vi "HAPS_LoadTable_SetBeam_Manual_Selected_Two_Phase.vi"() -> ()   [LabVIEW 2023, in "HAPS.lvlib"]
uses:
  HAPS.lvlib
  set_ele.ctl
  HAPS_SerialPort.ctl
  HAPS_MCU_ELE_Func.ctl
  <vilib>/Utility/file.llb/Read Delimited Spreadsheet (string).vi
  R_S/R_S.lvlib
panel:
  in  "Phase_offset?":i32
  in  "ele_gain_2":i32=35
  in  "BFIC_id_2?":i32
  in  "Group_2?":i32
  in  "ele_gain_1":i32=35
  in  "BFIC_id_1?":i32
  in  "Group_1?":i32
  in  "sys reboot?":bool=TRUE
  in  "VISA resource name":refnum<visa-resource-name>="COM1"
  in  "file path":path=path "D:/_Project/_Code/LabVIEW/_CLC_Gen4/CLC_LV2023/CLC_Cali/Log/HAPS/Preset.csv"
  out "error IO":errorcluster
  out "Err_code":i32
  out "status":bool
  in  "simu.?":bool
  in  "set_ele":T1={"ch"=0, "chain_id"=0, "group"=0, "array_id"=0, "ele_phase"=0, "ele_gain"=35, "com_gain"=17, "pd_range"=0}
  out "ele phase":i32
  out "ele gain":i32
  out "channel":i32
  out "chain ID":i32
  out "group":i32
  out "array id":i32
  # "HAPS 24x24 Setting Manual In-Phase : \n                                           Two BFIC Phase"
  # "Tx:35\nRx:22"
  # "Not using!!!!!!!!!!!!!!!!!!!!!!!!!!!!!!!!!!!!!!!!"
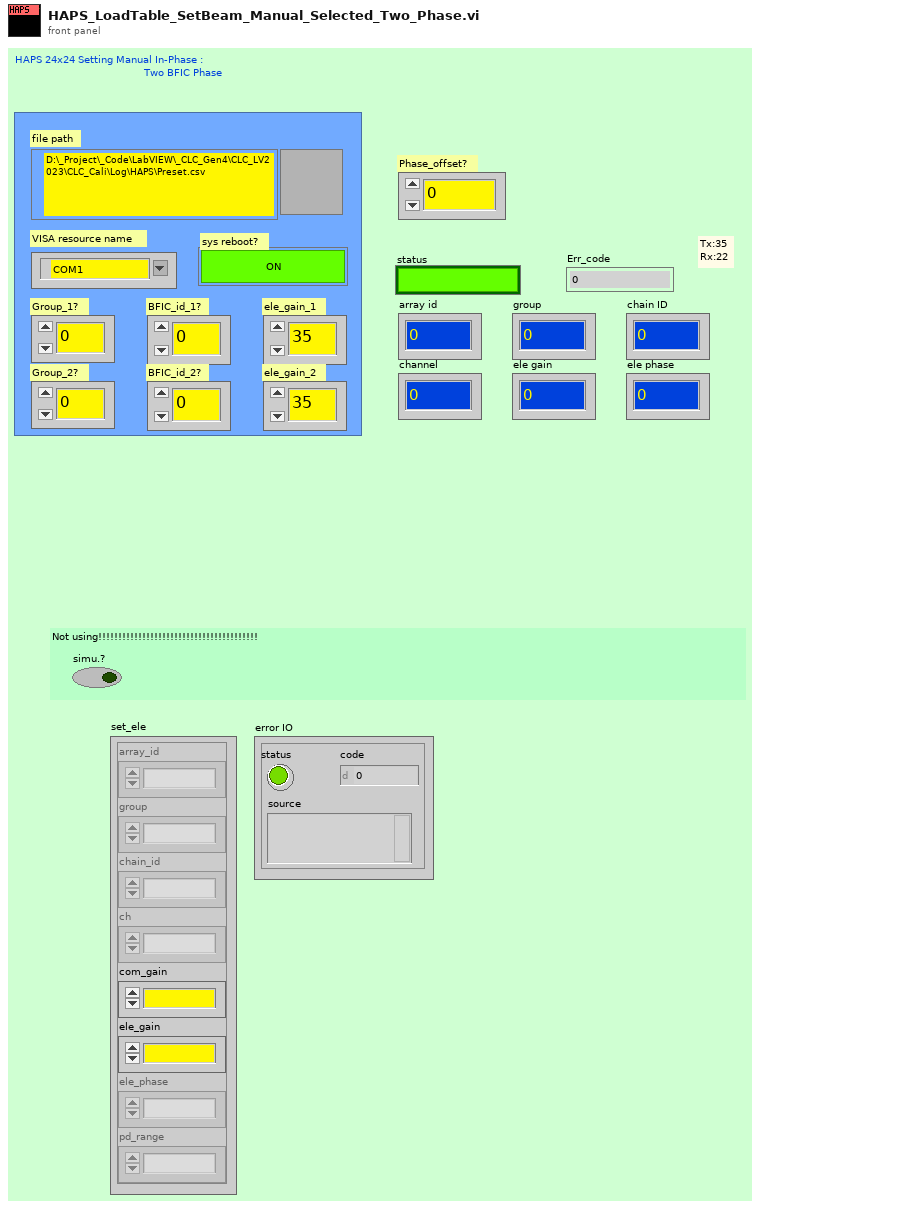
[diagram p1: front panel]
types:
  T1 = typedef "HAPS.lvlib/set_ele.ctl" = cluster{"ch":i32, "chain_id":i32, "group":i32, "array_id":i32, "ele_phase":i32, "ele_gain":i32, "com_gain":i32, "pd_range":i32}
  T2 = typedef "HAPS.lvlib/HAPS_SerialPort.ctl" = enum16{"Init", "Close", "CMD", "Flush"}
  T3 = typedef "HAPS.lvlib/HAPS_MCU_ELE_Func.ctl" = enum16{"array_init", "set_com_gain", "set_ch_gain_phase", "set_pd_range", "get_preamp_temp", "get_bfic_temp", "get_tx_pd", "ch_on", "ch_on_2", "ch_ctrl_all", "array_ctrl_src"}
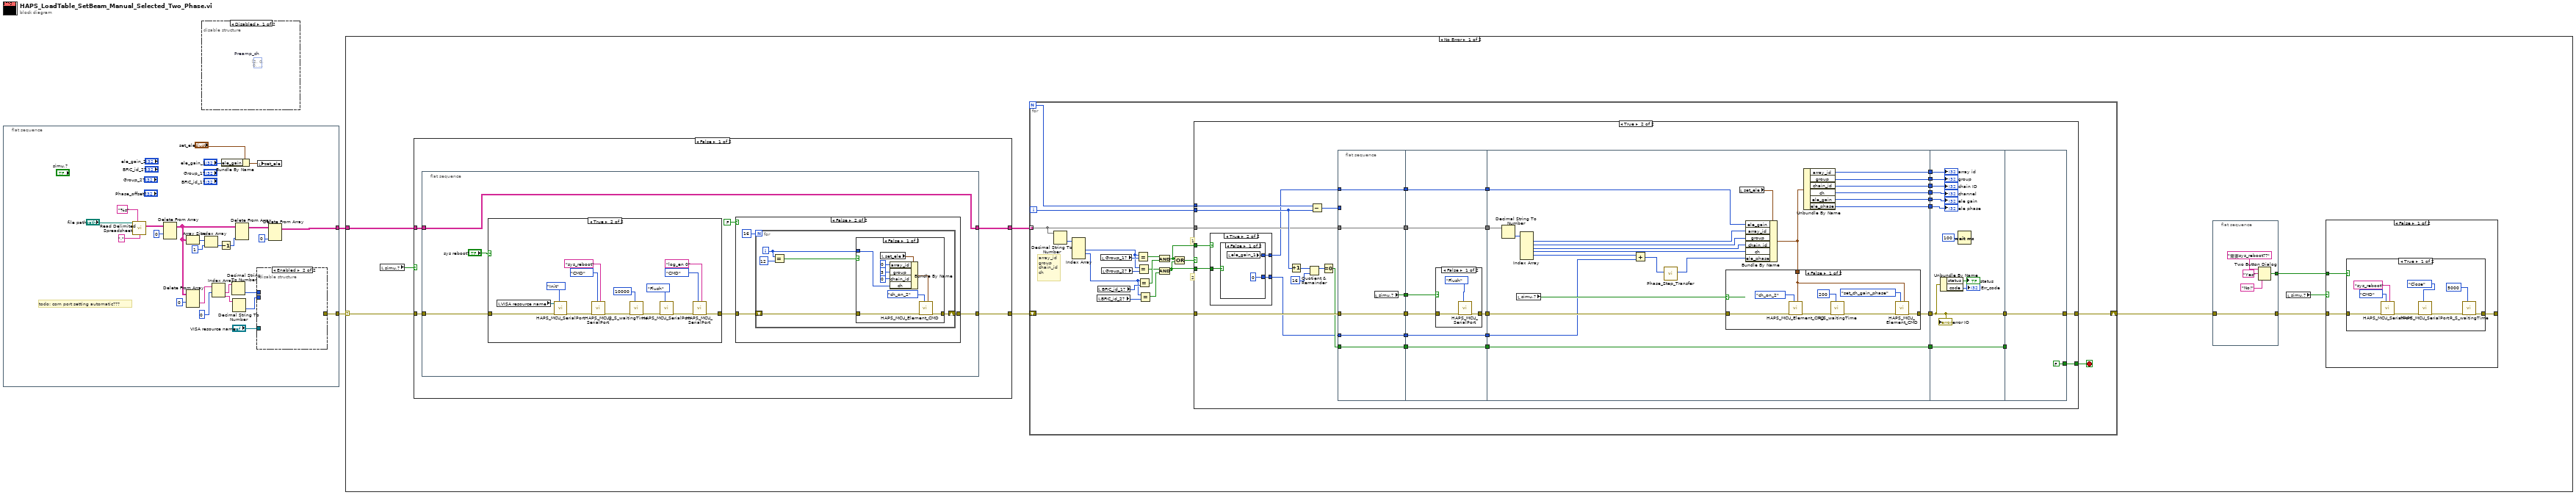
[diagram p0: block diagram]
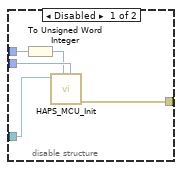
[diagram p2: hidden frame]
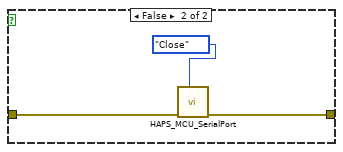
[diagram p4: hidden frame]
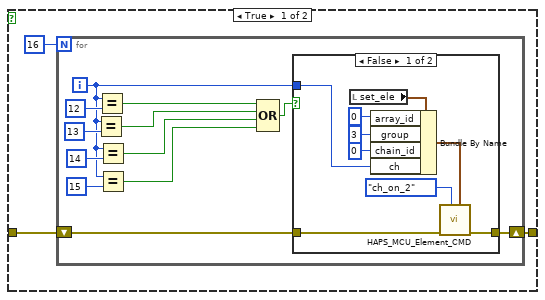
[diagram p6: hidden frame]
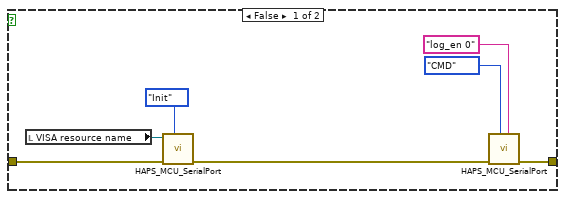
[diagram p9: hidden frame]
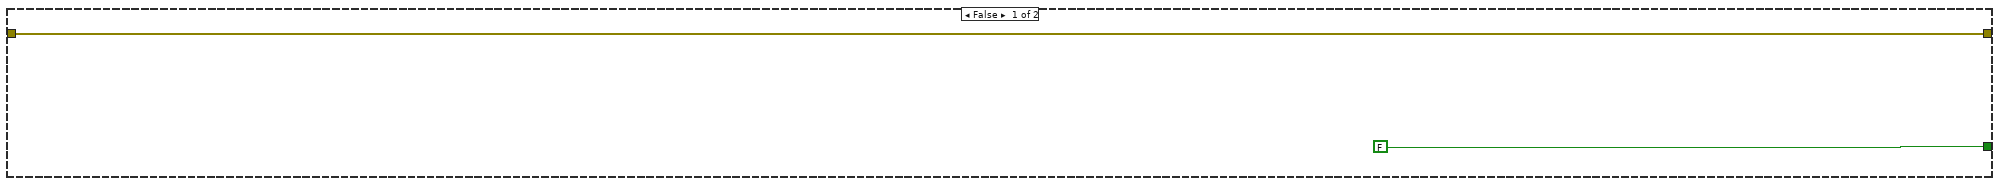
[diagram p11: hidden frame]
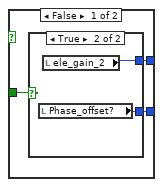
[diagram p12: hidden frame]
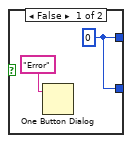
[diagram p13: hidden frame]
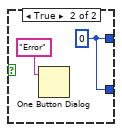
[diagram p14: hidden frame]
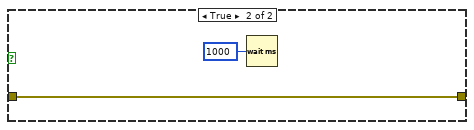
[diagram p16: hidden frame]
diagram:
  n1 = flat-sequence {
    tunnel: [w19] -> w2
    tunnel: [w6] -> w1
    frame #0 {
      # "todo: com port setting automatic???"
      n2 = call-poly <vilib>:"Read Delimited Spreadsheet.vi"("file path (dialog if empty)"="file path", "format (%s)"="%s" ("format (%.3f)"), "delimiter (\\t)"="," ("delimiter (\\t)")) -> ("all rows"=w25:string[][])  [unwired: 7 in, 5 out]
      n3 = Delete From Array(array=w25, index (row)=0) -> (array with subset deleted=w15:string[][])  [unwired: 2 in, 1 out]
      n4 = Array Size(array=w15) -> (size(s)=w23:i32[])
      n5 = Delete From Array(array=w15, index (row)=0) -> (deleted portion=w14:string[])  [unwired: 2 in, 1 out]
      n6 = Index Array(array=w23, index=1) -> (element=w20:i32)
      n7 = Index Array(array=w14, index #1=0 ("index")) -> (element #1=w13:string, element #2=w12:string)  [unwired: 1 in]
      n8 = Decrement(x=w20) -> (x-1=w22:i32)
      n9 = Bundle By Name(cluster="set_ele", "ele_gain"="ele_gain_1") -> (w3:T1)
      n10 = Decimal String To Number(string=w13) -> (number=w9:i32)  [unwired: 2 in, 1 out]
      n11 = Decimal String To Number(string=w12) -> (number=w8:i32)  [unwired: 2 in, 1 out]
      n12 = Delete From Array(array=w15, index (col)=w22) -> (array with subset deleted=w18:string[][])  [unwired: 2 in, 1 out]
      n13 = disable-structure shown="Enabled" {
        disable-tunnel: [w32 _] -> w19
        disable-tunnel: w9 -> [w31 _]
        disable-tunnel: w8 -> [w30 _]
        disable-tunnel: "VISA resource name" -> [w29 _]
        frame Disabled {
          n14 = To Unsigned Word Integer(number=w31) -> (unsigned 16bit integer=w28:u16)
          n15 = call "HAPS_MCU_Init.vi"("array_id"=w30, "Tx/Rx"=w28, "VISA resource name"=w29) -> ("error out"=w32:errorcluster)  [unwired: 8 in]
        }
        frame Enabled {
        }
      }
      n16 = local write "set_ele"(w3) -> ()
      n17 = Delete From Array(array=w18, index (col)=0 ("index (row)")) -> (array with subset deleted=w6:string[][])  [unwired: 2 in, 1 out]
    }
  }
  n18 = disable-structure shown="Disabled" {
    frame Disabled {
      (unwired) i32[][] [[2, 0, 0, 8, 8, 10, 11, 9, 9, 1, 1, 3], [3, 1, 1, 9, 9, 11, 13, 15, 15, 7, 7, 5], [5, 7, 7, 15, 15, 13, 14, 14, 6, 6, 4, 12]]  # Preamp_ch
    }
    frame Enabled {
    }
  }
  n19 = case shown="No Error" w2 {
    selector: w2 -> [w39 _]
    tunnel: w1 -> [w41 _]
    frame No Error {
      n20 = local read "simu.?"() -> (w37:bool)
      n21 = case shown="False" w37 {
        tunnel: w41 -> [w65 w137]
        tunnel: [w64 w137] -> w40
        tunnel: w39 -> [w63 w136]
        tunnel: [w62 w136] -> w38
        frame False {
          n22 = flat-sequence {
            tunnel: w65 -> [w71]
            tunnel: [w71] -> w64
            tunnel: w63 -> [w69]
            tunnel: [w70] -> w62
            frame #0 {
              n23 = case shown="True" "sys reboot?" {
                tunnel: w69 -> [w119 w133]
                tunnel: [w117 w131] -> w68
                frame False {
                  n24 = local read "VISA resource name"() -> (w115:refnum<visa-resource-name>)
                  n25 = call "HAPS_MCU_SerialPort.vi"("HAPS_SerialPort_Func"=HAPS_SerialPort."Init", "error in"=w119, "VISA resource name"=w115) -> ("error out"=w116:errorcluster)  [unwired: 6 in, 2 out]
                  n26 = call "HAPS_MCU_SerialPort.vi"("Command"="log_en 0", "HAPS_SerialPort_Func"=enum16{"Init", "Close", "CMD"}."CMD" ("HAPS_SerialPort"), "error in"=w116) -> ("error out"=w117:errorcluster)  [unwired: 6 in, 2 out]
                }
                frame True {
                  n27 = local read "VISA resource name"() -> (w122:refnum<visa-resource-name>)
                  n28 = call "HAPS_MCU_SerialPort.vi"("HAPS_SerialPort_Func"=HAPS_SerialPort."Init", "error in"=w133, "VISA resource name"=w122) -> ("error out"=w128:errorcluster)  [unwired: 6 in, 2 out]
                  n29 = call "HAPS_MCU_SerialPort.vi"("Command"="sys_reboot", "HAPS_SerialPort_Func"=enum16{"Init", "Close", "CMD"}."CMD" ("HAPS_SerialPort"), "error in"=w128) -> ("error out"=w127:errorcluster)  [unwired: 6 in, 2 out]
                  n30 = call "R_S_waitingTime.vi"("Waiting Time(ms)"=u32 10000, "error in"=w127) -> ("error out"=w125:errorcluster)  [unwired: 9 in]
                  n31 = call "HAPS_MCU_SerialPort.vi"("HAPS_SerialPort_Func"=HAPS_SerialPort."Flush", "error in"=w125) -> ("error out"=w123:errorcluster)  [unwired: 7 in, 2 out]
                  n32 = call "HAPS_MCU_SerialPort.vi"("Command"="log_en 0", "HAPS_SerialPort_Func"=enum16{"Init", "Close", "CMD"}."CMD" ("HAPS_SerialPort"), "error in"=w123) -> ("error out"=w131:errorcluster)  [unwired: 6 in, 2 out]
                }
              }
              n33 = case shown="False" FALSE {
                tunnel: [w73 w98] -> w70
                tunnel: w68 -> [w72 w97]
                frame True {
                  n34 = for {
                    N: 16 -> [_]
                    shift-right: [w85] -> w73
                    shift-left: w72 -> [w86]
                    i -> [w76]
                    n35 = Equal?(x=w76, y=13) -> (x = y?=w80:bool)
                    n36 = Equal?(x=w76, y=12) -> (x = y?=w84:bool)
                    n37 = Equal?(x=w76, y=14) -> (x = y?=w78:bool)
                    n38 = Equal?(x=w76, y=15) -> (x = y?=w75:bool)
                    n39 = Compound Arithmetic op=OR(w84, w80, w78, w75) -> (w81:bool)
                    n40 = case shown="False" w81 {
                      tunnel: w86 -> [w89 w96]
                      tunnel: [w88 w96] -> w85
                      tunnel: w76 -> [w87 _]
                      frame False {
                        n41 = local read "set_ele"() -> (w91:T1)
                        n42 = Bundle By Name(cluster=w91, "array_id"=0, "group"=3, "chain_id"=0, "ch"=w87) -> (w92:T1)
                        n43 = call "HAPS_MCU_Element_CMD.vi"("set_ele"=w92, "HAPS_MCU_ELE_Func."=HAPS_MCU_ELE_Func."ch_on_2", "error in"=w89) -> ("error out"=w88:errorcluster)  [unwired: 7 in, 1 out]
                      }
                      frame True {
                      }
                    }
                  }
                }
                frame False {
                  n44 = for {
                    N: 16 -> [_]
                    shift-right: [w103] -> w98
                    shift-left: w97 -> [w104]
                    i -> [w101]
                    n45 = Equal?(x=w101, y=12) -> (x = y?=w100:bool)
                    n46 = case shown="False" w100 {
                      tunnel: w104 -> [w107 w114]
                      tunnel: [w106 w114] -> w103
                      tunnel: w101 -> [w105 _]
                      frame False {
                        n47 = local read "set_ele"() -> (w109:T1)
                        n48 = Bundle By Name(cluster=w109, "array_id"=0, "group"=3, "chain_id"=0, "ch"=w105) -> (w110:T1)
                        n49 = call "HAPS_MCU_Element_CMD.vi"("set_ele"=w110, "HAPS_MCU_ELE_Func."=HAPS_MCU_ELE_Func."ch_on_2", "error in"=w107) -> ("error out"=w106:errorcluster)  [unwired: 7 in, 1 out]
                      }
                      frame True {
                      }
                    }
                  }
                }
              }
            }
          }
        }
        frame True {
        }
      }
      n50 = for {
        N -> [w155]
        tunnel: w40 -> [w152] mode=indexing
        shift-right: [w157] -> w34
        shift-left: w38 -> [w156]
        i -> [w154]
        stop <- w151 stop-if-true
        # "2"
        # "1"
        # "array_id\ngroup\nchain_id\nch"
        n51 = Decimal String To Number(string=w152) -> (number=w153:i32[])  [unwired: 2 in, 1 out]
        n52 = Index Array(array=w153) -> (element #2=w147:i32, element #3=w144:i32)  [unwired: 4 in, 2 out]
        n53 = local read "BFIC_id_2?"() -> (w143:i32)
        n54 = local read "BFIC_id_1?"() -> (w145:i32)
        n55 = local read "Group_1?"() -> (w148:i32)
        n56 = local read "Group_2?"() -> (w146:i32)
        n57 = Equal?(x=w147, y=w148) -> (x = y?=w150:bool)
        n58 = Equal?(x=w147, y=w146) -> (x = y?=w142:bool)
        n59 = Equal?(x=w144, y=w145) -> (x = y?=w149:bool)
        n60 = Equal?(x=w144, y=w143) -> (x = y?=w141:bool)
        n61 = Compound Arithmetic op=AND(w150, w149) -> (w139:bool)
        n62 = Compound Arithmetic op=AND(w142, w141) -> (w138:bool)
        n63 = Compound Arithmetic op=OR(w139, w138) -> (w140:bool)
        n64 = case shown="True" w140 {
          tunnel: [w158 w179] -> w157
          tunnel: w156 -> [w158 w178]
          tunnel: w155 -> [_ w177]
          tunnel: w154 -> [_ w176]
          tunnel: w152 -> [_ w175]
          tunnel: [FALSE ("T button?") w169] -> w151
          tunnel: w139 -> [_ w167]
          tunnel: w138 -> [_ w166]
          frame False {
          }
          frame True {
            n65 = case shown="True" w167 {
              tunnel: w166 -> [w198 w204]
              tunnel: [w197 w205] -> w163
              tunnel: [w196 w203] -> w160
              frame False {
                n66 = case shown="True" w198 {
                  tunnel: [w199 w202] -> w197
                  tunnel: [w199 w201] -> w196
                  frame False {
                    w199 = 0 ("ele_gain_2")
                    n67 = One Button Dialog(message="Error") -> ()  [unwired: 1 in, 1 out]
                  }
                  frame True {
                    n68 = local read "Phase_offset?"() -> (w201:i32)
                    n69 = local read "ele_gain_2"() -> (w202:i32)
                  }
                }
              }
              frame True {
                n70 = case shown="False" w204 {
                  tunnel: [w207 w208] -> w205
                  tunnel: [0 ("ele_gain_2") w208] -> w203
                  frame False {
                    n71 = local read "ele_gain_1"() -> (w207:i32)
                  }
                  frame True {
                    w208 = 0 ("ele_gain_1")
                    n72 = One Button Dialog(message="Error") -> ()  [unwired: 1 in, 1 out]
                  }
                }
              }
            }
            n73 = Increment(x=w176) -> (x+1=w173:i32)
            n74 = Quotient & Remainder(x=w173, y=16) -> (x-y*floor(x/y)=w171:i32)  [unwired: 1 out]
            n75 = Subtract(x=w177, y=w176) -> (x-y=w174:i32)
            n76 = Equal To 0?(x=w171) -> (x = 0?=w170:bool)
            n77 = flat-sequence {
              tunnel: w174 -> [_]
              tunnel: w178 -> [w214]
              tunnel: w175 -> [w215]
              tunnel: [w215] -> w195
              tunnel: [w214] -> w194
              tunnel: w170 -> [w213]
              tunnel: [w213] -> w193
              tunnel: [w212] -> w168
              tunnel: [w211] -> w164
              tunnel: w163 -> [w211]
              tunnel: [w210] -> w161
              tunnel: w160 -> [w210]
              tunnel: [w222] -> w192
              tunnel: [w221] -> w191
              tunnel: w195 -> [w222]
              tunnel: w194 -> [w220]
              tunnel: w193 -> [w219]
              tunnel: [w219] -> w190
              tunnel: w168 -> [w218]
              tunnel: [w217] -> w165
              tunnel: w164 -> [w217]
              tunnel: [w216] -> w162
              tunnel: w161 -> [w216]
              tunnel: w192 -> [w249]
              tunnel: w191 -> [w247]
              tunnel: [w235] -> w189
              tunnel: [w245] -> w188
              tunnel: [w244] -> w187
              tunnel: [w243] -> w186
              tunnel: [w242] -> w185
              tunnel: [w241] -> w184
              tunnel: [w240] -> w183
              tunnel: w190 -> [w236]
              tunnel: [w236] -> w182
              tunnel: w165 -> [w231]
              tunnel: w162 -> [w229]
              tunnel: w189 -> [w262]
              tunnel: w188 -> [w270]
              tunnel: w187 -> [w269]
              tunnel: w186 -> [w268]
              tunnel: w185 -> [w267]
              tunnel: w184 -> [w266]
              tunnel: w183 -> [w265]
              tunnel: [w262] -> w181
              tunnel: w182 -> [w263]
              tunnel: [w263] -> w180
              tunnel: w181 -> [w272]
              tunnel: w180 -> [_]
              tunnel: [w272] -> w179
              tunnel: [FALSE ("T button?")] -> w169
              frame #0 {
                n78 = local read "simu.?"() -> (w212:bool)
              }
              frame #1 {
                n79 = case shown="False" w218 {
                  tunnel: [w225 w226] -> w221
                  tunnel: w220 -> [w224 w226]
                  frame False {
                    n80 = call "HAPS_MCU_SerialPort.vi"("HAPS_SerialPort_Func"=HAPS_SerialPort."Flush", "error in"=w224) -> ("error out"=w225:errorcluster)  [unwired: 7 in, 2 out]
                  }
                  frame True {
                  }
                }
              }
              frame #2 {
                n81 = Decimal String To Number(string=w249) -> (number=w248:i32[])  [unwired: 2 in, 1 out]
                n82 = local read "simu.?"() -> (w234:bool)
                n83 = Index Array(array=w248) -> (element #1=w246:i32, element #2=w239:i32, element #3=w238:i32, element #4=w232:i32, element #5=w230:i32)  [unwired: 6 in, 1 out]
                n84 = Add(x=w230, y=w229) -> (x+y=w228:i32)
                n85 = call "Phase_Step_Transfer.vi"("Input_Phase_Step"=w228) -> ("Output_Phase_Step"=w227:i32)  [unwired: 10 in]
                n86 = local read "set_ele"() -> (w237:T1)
                n87 = Bundle By Name(cluster=w237, "ele_gain"=w231, "array_id"=w246, "group"=w239, "chain_id"=w238, "ch"=w232, "ele_phase"=w227) -> (w233:T1)
                n88 = case shown="False" w234 {
                  tunnel: w247 -> [w257 w259]
                  tunnel: w233 -> [w256 _]
                  tunnel: [w255 w259] -> w235
                  frame False {
                    n89 = call "HAPS_MCU_Element_CMD.vi"("set_ele"=w256, "HAPS_MCU_ELE_Func."=HAPS_MCU_ELE_Func."ch_on_2", "error in"=w257) -> ("error out"=w251:errorcluster)  [unwired: 7 in, 1 out]
                    n90 = call "R_S_waitingTime.vi"("Waiting Time(ms)"=u32 200, "error in"=w251) -> ("error out"=w250:errorcluster)  [unwired: 9 in]
                    n91 = call "HAPS_MCU_Element_CMD.vi"("set_ele"=w256, "HAPS_MCU_ELE_Func."=HAPS_MCU_ELE_Func."set_ch_gain_phase", "error in"=w250) -> ("error out"=w255:errorcluster)  [unwired: 7 in, 1 out]
                  }
                  frame True {
                    n92 = Wait (ms)(milliseconds to wait=u32 1000) -> ()  [unwired: 1 out]
                  }
                }
                n93 = Unbundle By Name(w233) -> ("array_id"=w245:i32, "group"=w244:i32, "chain_id"=w243:i32, "ch"=w242:i32, "ele_gain"=w241:i32, "ele_phase"=w240:i32)
              }
              frame #3 {
                n94 = Unbundle By Name(w262) -> ("status"=→"status":bool, "code"=→"Err_code":i32)
                n95 = Wait (ms)(milliseconds to wait=u32 100) -> ()  [unwired: 1 out]
                "group" <- w269
                "chain ID" <- w268
                "channel" <- w267
                "ele gain" <- w266
                "ele phase" <- w265
                "array id" <- w270
                "error IO" <- w262
              }
              frame #4 {
              }
            }
          }
        }
      }
      n96 = flat-sequence {
        tunnel: w34 -> [w46]
        tunnel: [w46] -> w35
        tunnel: [w42] -> w36
        frame #0 {
          n97 = Two Button Dialog(message="需要sys_reboot??", 1:"No!" ("F button name (\"Cancel\")"), 2:"Yes" ("T button name (\"OK\")")) -> (T button?=w42:bool)
        }
      }
      n98 = local read "simu.?"() -> (w33:bool)
      n99 = case shown="False" w33 {
        tunnel: [w48 w61] -> _
        tunnel: w35 -> [w49 w61]
        tunnel: w36 -> [w47 _]
        frame False {
          n100 = case shown="True" w47 {
            tunnel: w49 -> [w57 w59]
            tunnel: [w50 w58] -> w48
            frame True {
              n101 = call "HAPS_MCU_SerialPort.vi"("Command"="sys_reboot", "HAPS_SerialPort_Func"=enum16{"Init", "Close", "CMD"}."CMD" ("HAPS_SerialPort"), "error in"=w57) -> ("error out"=w53:errorcluster)  [unwired: 6 in, 2 out]
              n102 = call "HAPS_MCU_SerialPort.vi"("HAPS_SerialPort_Func"=HAPS_SerialPort."Close", "error in"=w53) -> ("error out"=w51:errorcluster)  [unwired: 7 in, 2 out]
              n103 = call "R_S_waitingTime.vi"("Waiting Time(ms)"=u32 5000, "error in"=w51) -> ("error out"=w50:errorcluster)  [unwired: 9 in]
            }
            frame False {
              n104 = call "HAPS_MCU_SerialPort.vi"("HAPS_SerialPort_Func"=HAPS_SerialPort."Close", "error in"=w59) -> ("error out"=w58:errorcluster)  [unwired: 7 in, 2 out]
            }
          }
        }
        frame True {
        }
      }
    }
    frame Error {
    }
  }
